vi "Fetch Multiple Record Single Channel (I16).vi"(5 "FIFO Type":enum16{"FPGA to Host FIFO (U64)", "Generic"}(ring), 7 "Timeout (s)":i32=5, 8 "error in":errorcluster, 10 "Records to Fetch":i32, 11 "FPGA VI Reference In":refnum<k20>) -> (0 "error out":errorcluster, 2 "Acquired Data":i16[][](array[numeric]), 3 "FPGA VI Reference Out":refnum<k20>, 4 "Elements Remaining":u32)   [LabVIEW 2011]
uses:
  <userlib>/FlexRIO Host Library/FlexRIO Host API/Acquire/Fetch/Fetch Acquired Data (U64).vi
  <vilib>/Utility/error.llb/Error Cluster From Error Code.vi
  <vilib>/rvi/errors/niLvFpgaAdjustHostInterfaceError.vi
  <vilib>/rvi/interface/nirviReadWriteControl/nirviReadWriteControl.xnode
  NiFpgaLv.dll
  <vilib>/rvi/interface/Simulation/niFpgaSimulationCallBeginRW.vi
  <userlib>/FlexRIO Host Library/FlexRIO Host Library (User).lvlib
  <userlib>/FlexRIO Host Library/FlexRIO Host API/Utility/memnoncopy.dll
panel:
  out "Data Acquired":i16[](array[numeric])
  out "Dummy Data":i16[](array[numeric])
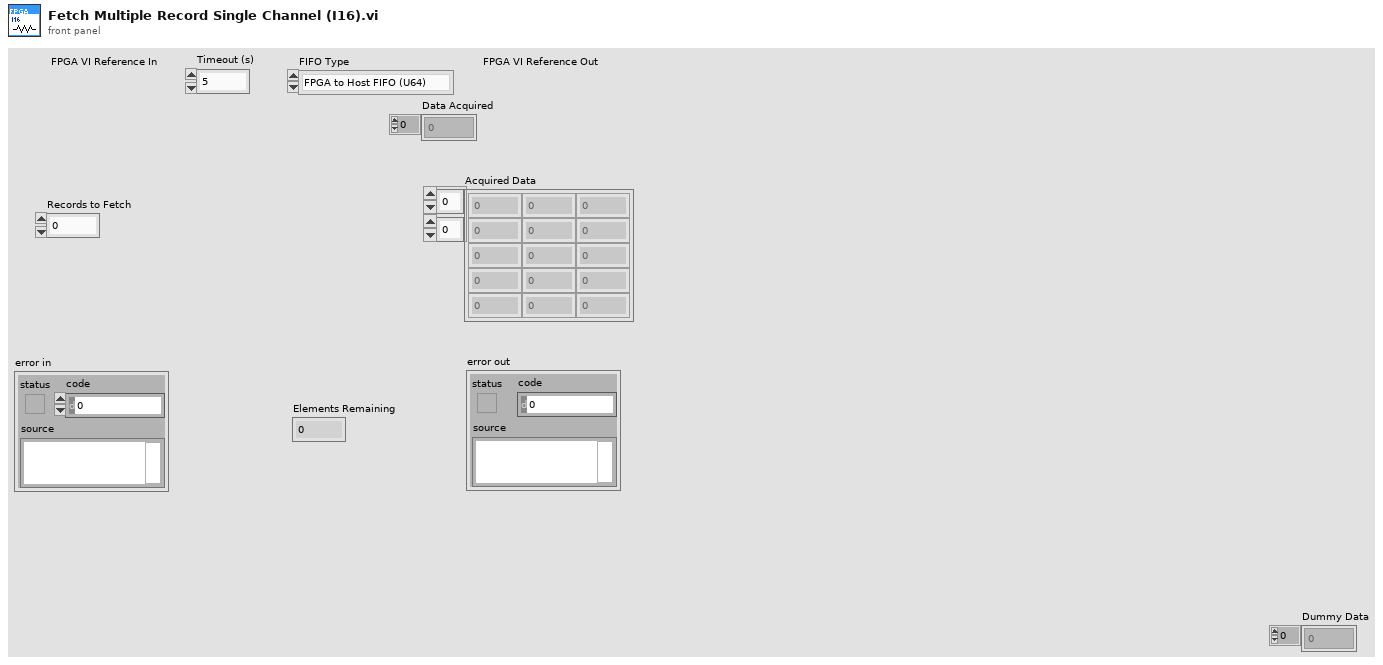
[diagram p1: front panel]
types:
  T1 = cluster{"Load Record Parameters?":bool, "Pre Trigger Samples":u16, "Samples per Record":u16, "Trigger Hold Off":u16, "Record Count":u16}
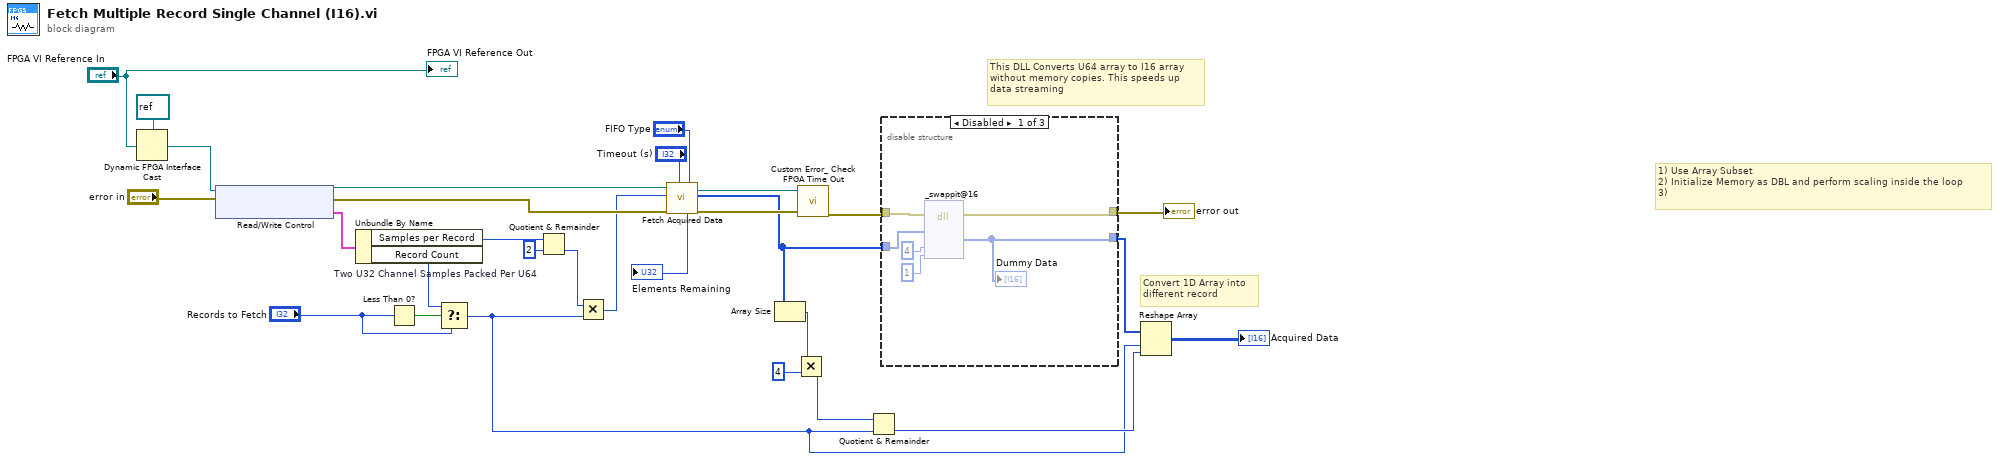
[diagram p0: block diagram]
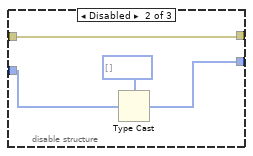
[diagram p2: hidden frame]
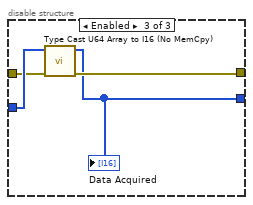
[diagram p3: hidden frame]
diagram:
  w12 = u16 2  # Two U32 Channel Samples Packed Per U64
  # "This DLL Converts U64 array to I16 array \nwithout memory copies. This speeds up \ndata streaming"
  # "Convert 1D Array into\ndifferent record"
  # "1) Use Array Subset\n2) Initialize Memory as DBL and perform scaling inside the loop\n3)"
  n1 = Dynamic FPGA Interface Cast(Session In=refnum<k20> refnum ("Type"), Type="FPGA VI Reference In") -> (Session Out=w26:refnum<k20>)
  n2 = xnode "Read/Write Control"("FPGA VI Reference In"=w26, "error in"="error in") -> ("FPGA VI Reference Out"=w21:refnum<k20>, "error out"=w20:errorcluster, "Record Parameters"=w25:T1)
  n3 = Unbundle By Name(w25) -> ("Samples per Record"=w13:u16, "Record Count"=w23:u16)
  n4 = Less Than 0?(x="Records to Fetch") -> (x < 0?=w24:bool)
  n5 = Select(t=w23, s=w24, f="Records to Fetch") -> (s? t:f=w2:i32)
  n6 = Quotient & Remainder(x=w13, y=w12) -> (floor(x/y)=w5:u16)  [unwired: 1 out]
  n7 = Multiply(x=w5, y=w2) -> (x*y=w14:i32)
  n8 = call-poly <userlib>:"Fetch Acquired Data.vi"("FIFO Type"="FIFO Type", "Timeout (s)"="Timeout (s)", "error out"=w20, "Samples"=w14, "FPGA VI Reference In"=w21) -> ("error out"=w15:errorcluster, "Data"=w7:u64[], "FPGA VI Reference Out"=w16:refnum<k20>, "Elements Remaining"=→"Elements Remaining":u32)  [unwired: 3 in]
  n9 = Array Size(array=w7) -> (size(s)=w8:i32)
  n10 = Multiply(x=w8, y=4) -> (x*y=w4:i32)
  n11 = call <userlib>:"Custom Error_ Check FPGA Time Out.vi"("error in"=w15, "FPGA VI Reference In"=w16) -> ("error out"=w10:errorcluster)  [unwired: 8 in, 1 out]
  n12 = Quotient & Remainder(x=w4, y=w2) -> (floor(x/y)=w6:i32)  [unwired: 1 out]
  n13 = disable-structure shown="Disabled" {
    disable-tunnel: w7 -> [w33 w38 w43]
    disable-tunnel: w10 -> [w32 w36 w42]
    disable-tunnel: [w31 w36 w41] -> w9
    disable-tunnel: [w30 w37 w40] -> w1
    frame Disabled {
      n14 = dll-call lib="C:/Program Files (x86)/National Instruments/LabVIEW 2011/user.lib/FlexRIO Host Library/FlexRIO Host API/Utility/memnoncopy.dll" fn="_swappit@16"(error in=w32, "src"=w33, "upsize"=4, "downsize"=1) -> (error out=w31:errorcluster, "Dummy Data"=w30:i16[])  [unwired: 7 in, 1 out]
      "Dummy Data" <- w30
    }
    frame Disabled {
      n15 = Type Cast(type=i16[] [], x=w38) -> (*(type *) &x=w37:i16[])
    }
    frame Enabled {
      n16 = call <userlib>:"Type Cast U64 Array to I16 (No MemCpy).vi"("error in"=w42, "Input"=w43) -> ("error out"=w41:errorcluster, "Data Acquired"=w40:i16[])  [unwired: 8 in]
      "Data Acquired" <- w40
    }
  }
  "error out" <- w9
  n17 = Reshape Array(w1, w2, w6) -> (→"Acquired Data":i16[][])
  "FPGA VI Reference Out" <- "FPGA VI Reference In"
